vi "Convert-ImageJ-2017.vi"(11 "Error in":errorcluster) -> (4 "Results":string, 15 "Error out":errorcluster)   [LabVIEW 2020]
doc: "VI devoloped at University of Twente, BioPhysical Engineering, used for running ImageJ in LabVIEW. Insert the macro to be run in the top string. Make sure the macro is in the C:\\Program Files\\ImageJ directory."
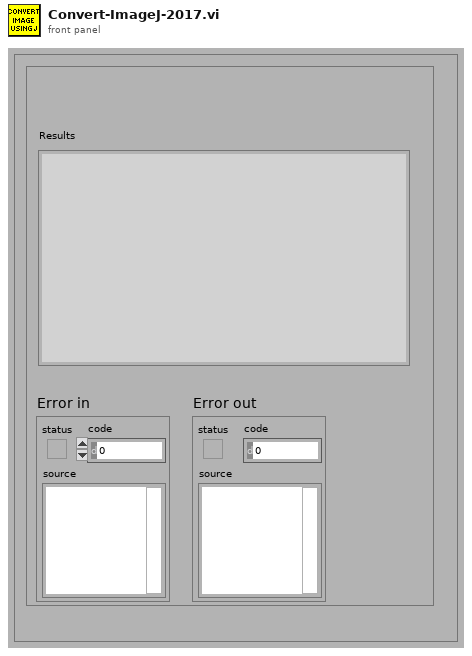
[diagram p1: front panel]
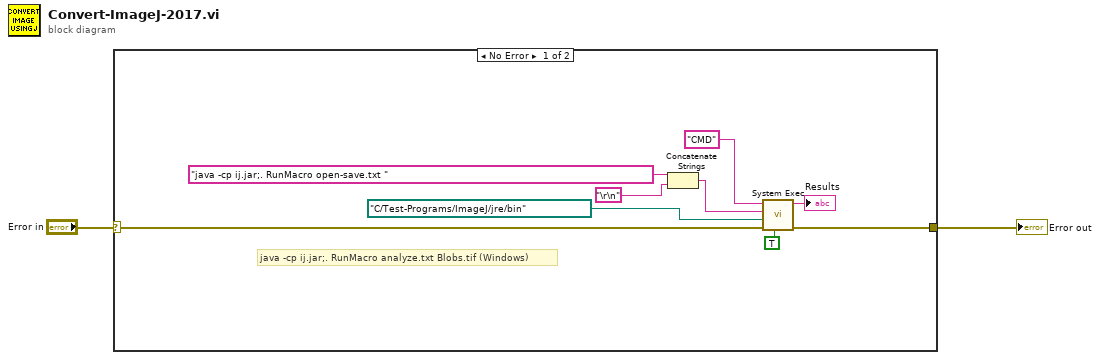
[diagram p0: block diagram]
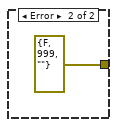
[diagram p2: hidden frame]
diagram:
  n1 = case shown="No Error" "Error in" {
    selector: "Error in" -> [w4 _]
    tunnel: [w3 errorcluster {"status"=FALSE, "code"=999, "source"=""} ("error out")] -> w1
    frame No Error {
      # "java -cp ij.jar;. RunMacro analyze.txt Blobs.tif (Windows)"
      n2 = Concatenate Strings("java -cp ij.jar;. RunMacro open-save.txt ", "\r\n") -> (w5:string)
      n3 = call <vilib>:"System Exec.vi"("run minimized? (F)"=TRUE, "error in (no error)"=w4, "working directory"=path "C:/Test-Programs/ImageJ/jre/bin", "standard input"=w5, "command line"="CMD") -> ("error out"=w3:errorcluster, "standard output"=→"Results":string)  [unwired: 3 in, 2 out]
    }
    frame Error {
    }
  }
  "Error out" <- w1
